vi "Set Actuator Set Points.vi"(10 "Actuator Set Points":T1 {"Lateral Force" format="%.4f"; "Axial Force" format="%.4f"; "FC2 Force" format="%.4f"; "FC1 Force" format="%.4f"}, 11 "Model in":refnum<class "Model.lvclass">) -> (3 "Model out":refnum<class "Model.lvclass">)   [LabVIEW 2016]
uses:
  Model.lvclass
  Typedefs/ActuatorSetPoints.ctl
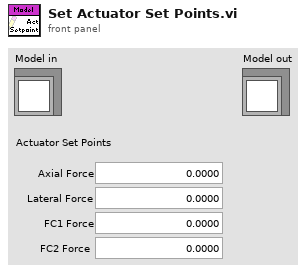
[diagram p1: front panel]
types:
  T1 = typedef "ActuatorSetPoints.ctl" = cluster{"Axial Force":dbl, "Lateral Force":dbl, "FC1 Force":dbl, "FC2 Force":dbl}
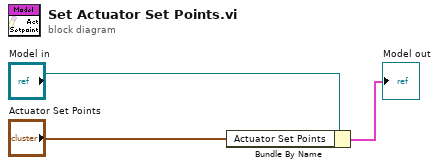
[diagram p0: block diagram]
diagram:
  n1 = Bundle By Name(cluster="Model in", "Actuator Set Points"="Actuator Set Points") -> (→"Model out":cluster{})
